vi "SMD7615 UDP Test.vi"() -> ()   [LabVIEW 2016, in "SMD-7615.lvlib" / "eSCL.lvlib"]
uses:
  eSCL.lvlib
panel:
  out "Move Complete":bool
  out "Input Status":string
  out "Velocity":i32
  out "Encoder":i32
  out "CCW Limit":bool
  out "CW Limit":bool
  in  "Distance / Position":i32
  in  "Move Mode":string
  in  "Reset Pos Button":bool
  in  "DAQ Button":bool
  in  "Move Button":bool
  in  "Stop Button":bool
  in  "Close ?":bool
  in  "Init ?":bool
  in  "Stop App":bool
  out "error out":errorcluster
  in  "address":string="192.168.1.30"
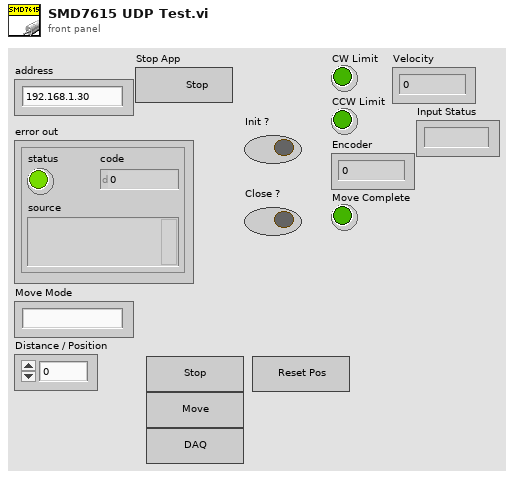
[diagram p1: front panel]
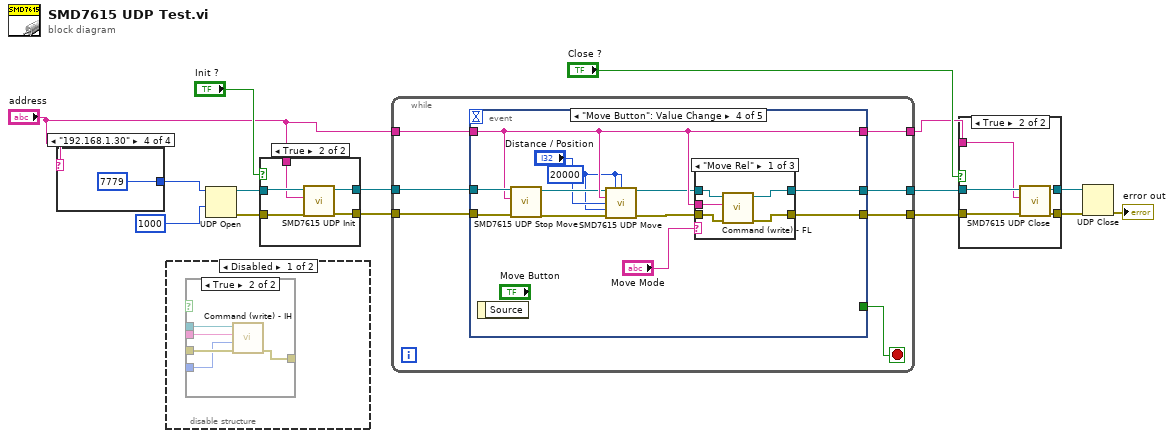
[diagram p0: block diagram]
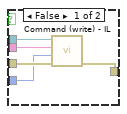
[diagram p2: hidden frame]
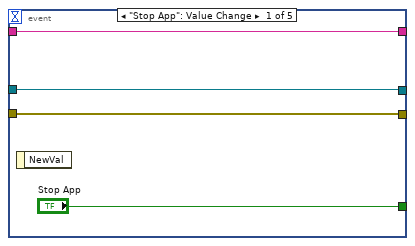
[diagram p4: hidden frame]
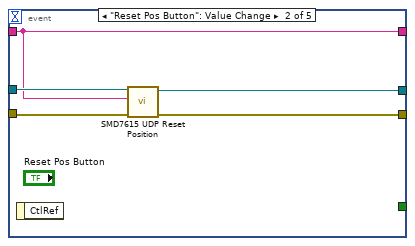
[diagram p5: hidden frame]
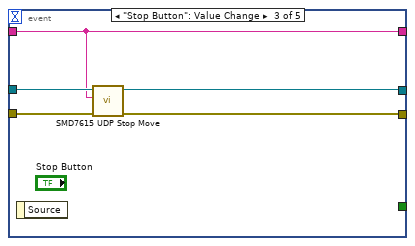
[diagram p6: hidden frame]
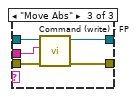
[diagram p8: hidden frame]
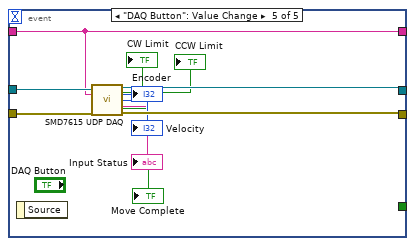
[diagram p9: hidden frame]
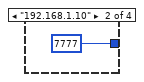
[diagram p13: hidden frame]
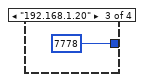
[diagram p14: hidden frame]
diagram:
  n1 = case shown="\"192.168.1.30\"" "address" {
    tunnel: [_ u16 7777 ("port") u16 7778 ("port") u16 7779 ("port")] -> w13
    frame "False", Default {
    }
    frame "192.168.1.10" {
    }
    frame "192.168.1.20" {
    }
    frame "192.168.1.30" {
    }
  }
  n2 = disable-structure shown="Disabled" {
    frame Disabled {
      n3 = case shown="True" {
        selector: _ -> [_ _]
        tunnel: _ -> [w22 w28]
        tunnel: _ -> [w21 w27]
        tunnel: _ -> [w20 w26]
        tunnel: [w23 w25] -> _
        tunnel: _ -> [w19 w24]
        frame False {
          n4 = call "Command (write) - IL.vi"("error in (no error)"=w21, "Output"=w20, "IP"=w19, "connection ID in"=w22) -> ("error out"=w23:errorcluster)  [unwired: 6 in, 1 out]
        }
        frame True {
          n5 = call "Command (write) - IH.vi"("error in (no error)"=w27, "Output"=w26, "IP"=w24, "connection ID in"=w28) -> ("error out"=w25:errorcluster)  [unwired: 6 in, 1 out]
        }
      }
    }
    frame Enabled {
    }
  }
  n6 = UDP Open(9:1000 ("timeout ms (25000)"), 11:w13) -> (port=w12:refnum<k16>, 0:w11:errorcluster)  [unwired: 3 in, 1 out]
  n7 = case shown="True" "Init ?" {
    tunnel: w12 -> [w30 w35]
    tunnel: w11 -> [w29 w34]
    tunnel: [w30 w33] -> w6
    tunnel: [w29 w32] -> w5
    tunnel: "address" -> [_ w31]
    frame False {
    }
    frame True {
      n8 = call "SMD7615 UDP Init.vi"("error in (no error)"=w34, "IP"=w31, "connection ID in"=w35) -> ("error out"=w32:errorcluster, "connection ID out"=w33:refnum<k16>)  [unwired: 7 in]
    }
  }
  n9 = while {
    tunnel: w6 -> [w41]
    tunnel: w5 -> [w40]
    tunnel: [w39] -> w4
    tunnel: [w38] -> w3
    tunnel: "address" -> [w37]
    tunnel: [w36] -> w1
    stop <- w42 stop-if-true
    n10 = event shown="[3] \"Move Button\": Value Change" {
      selector: _ -> [_ _ _ _ _]
      dyn-events: _ -> [_ _ _ _ _]
      timeout: _ -> [_ _ _ _ _]
      tunnel: ["Stop App" _ _ _ _] -> w42
      tunnel: w41 -> [w45 w51 w56 w68 w91]
      tunnel: w40 -> [w44 w50 w55 w67 w90]
      tunnel: [w44 w49 w52 w63 w87] -> w39
      tunnel: [w45 w48 w53 w62 w88] -> w38
      tunnel: w37 -> [w43 w47 w54 w65 w89]
      tunnel: [w43 w47 w54 w65 w89] -> w36
      event "Stop App": Value Change {
        n11 = event-data() -> ()  [unwired: 1 in, 1 out]
      }
      event "Reset Pos Button": Value Change {
        n12 = event-data() -> ()  [unwired: 1 in, 1 out]
        n13 = call "SMD7615 UDP Reset Position.vi"("error in (no error)"=w50, "IP"=w47, "connection ID in"=w51) -> ("error out"=w49:errorcluster, "connection ID out"=w48:refnum<k16>)  [unwired: 7 in]
      }
      event "Stop Button": Value Change {
        n14 = event-data() -> ()  [unwired: 1 in, 1 out]
        n15 = call "SMD7615 UDP Stop Move.vi"("error in (no error)"=w55, "IP"=w54, "connection ID in"=w56) -> ("error out"=w52:errorcluster, "connection ID out"=w53:refnum<k16>)  [unwired: 7 in]
      }
      event "Move Button": Value Change {
        w57 = 20000 ("Acceleration")
        n16 = event-data() -> ()  [unwired: 1 in, 1 out]
        n17 = call "SMD7615 UDP Stop Move.vi"("error in (no error)"=w67, "IP"=w65, "connection ID in"=w68) -> ("error out"=w60:errorcluster, "connection ID out"=w59:refnum<k16>)  [unwired: 7 in]
        n18 = call "SMD7615 UDP Move.vi"("connection ID in"=w59, "Acceleration"=w57, "Deceleration"=w57, "IP"=w65, "Distance / Position"="Distance / Position", "Velocity"=w57, "error in (no error)"=w60) -> ("connection ID out"=w64:refnum<k16>, "error out"=w61:errorcluster)  [unwired: 7 in]
        n19 = case shown="\"Move Rel\"" "Move Mode" {
          tunnel: w61 -> [w73 w75 w80]
          tunnel: w65 -> [w69 _ w76]
          tunnel: [w72 w74 w79] -> w62
          tunnel: [w71 w75 w78] -> w63
          tunnel: w64 -> [w70 w74 w77]
          frame "Move Rel" {
            n20 = call "Command (write) - FL.vi"("error in (no error)"=w73, "IP"=w69, "connection ID in"=w70) -> ("error out"=w71:errorcluster, "connection ID out"=w72:refnum<k16>)  [unwired: 7 in]
          }
          frame Default {
          }
          frame "Move Abs" {
            n21 = call "Command (write) - FP.vi"("error in (no error)"=w80, "IP"=w76, "connection ID in"=w77) -> ("error out"=w78:errorcluster, "connection ID out"=w79:refnum<k16>)  [unwired: 7 in]
          }
        }
      }
      event "DAQ Button": Value Change {
        n22 = event-data() -> ()  [unwired: 1 in, 1 out]
        n23 = call "SMD7615 UDP DAQ.vi"("connection ID in"=w91, "IP"=w89, "error in (no error)"=w90) -> ("CW Limit"=→"CW Limit":bool, "CCW Limit"=→"CCW Limit":bool, "connection ID out"=w88:refnum<k16>, "Encoder"=→"Encoder":i32, "Velocity"=→"Velocity":i32, "Input Status"=→"Input Status":string, "Move Complete"=→"Move Complete":bool, "error out"=w87:errorcluster)  [unwired: 5 in]
      }
    }
  }
  n24 = case shown="True" "Close ?" {
    tunnel: [w92 w98] -> w10
    tunnel: [w93 w97] -> w9
    tunnel: w4 -> [w92 w96]
    tunnel: w3 -> [w93 w95]
    tunnel: w1 -> [_ w94]
    frame False {
    }
    frame True {
      n25 = call "SMD7615 UDP Close.vi"("error in (no error)"=w96, "IP"=w94, "connection ID in"=w95) -> ("error out"=w98:errorcluster, "connection ID out"=w97:refnum<k16>)  [unwired: 7 in]
    }
  }
  n26 = UDP Close(connection ID=w9, 8:w10) -> (error out=→"error out":errorcluster)  [unwired: 1 out]
